vi "generate-uhd-class-lib.vi"() -> ()   [LabVIEW 2023]
panel:
  out "error out":errorcluster
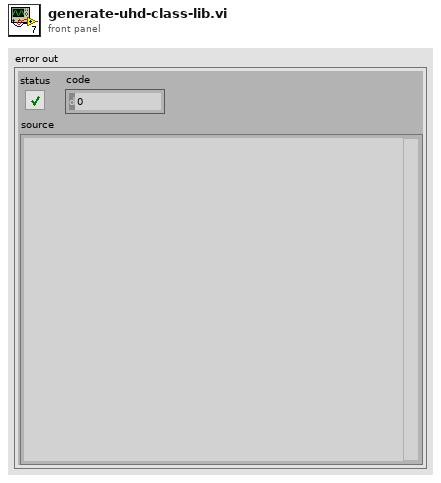
[diagram p1: front panel]
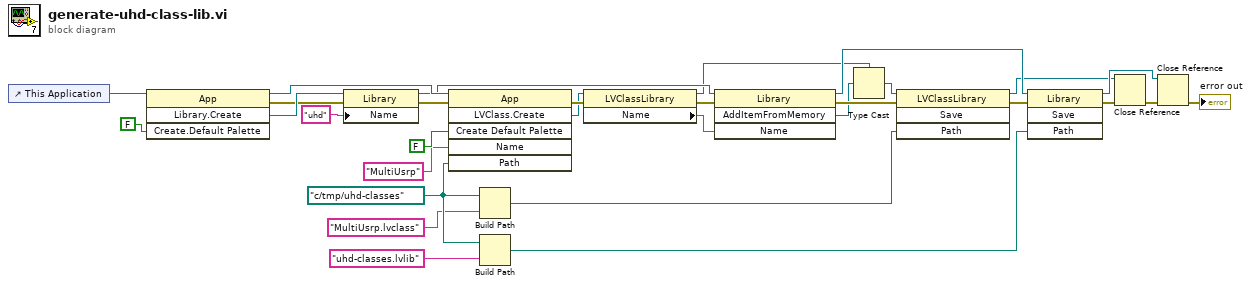
[diagram p0: block diagram]
diagram:
  w15 = path "c:/tmp/uhd-classes"
  n1 = control-ref of="This Application"() -> (w30:refnum<vi>)
  n2 = invoke class="App" method="Library.Create"(reference=w30, "Create.Default Palette"=FALSE ("Create:Default Palette")) -> (reference out=w28:refnum<vi>, error out=w21:errorcluster, "Create Library"=w23:refnum<vi>)  [unwired: 2 in, 1 out]
  n3 = property class="Library"(reference=w23, error in=w21, "Name"="uhd") -> (reference out=w13:refnum<vi>, error out=w20:errorcluster)
  n4 = invoke class="App" method="LVClass.Create"(reference=w28, error in=w20, "Create Default Palette"=FALSE ("Create:Default Palette"), "Name"="MultiUsrp", "Path"=w15) -> (error out=w11:errorcluster, "LVClass.Create"=w1:refnum<vi>)  [unwired: 1 in, 4 out]
  n5 = Build Path(base path=w15, name or relative path="MultiUsrp.lvclass" ("Name")) -> (appended path=w9:path)
  n6 = Build Path(base path=w15, name or relative path="uhd-classes.lvlib" ("Name")) -> (appended path=w16:path)
  n7 = property class="LVClassLibrary"(reference=w1, error in=w11) -> (reference out=w3:refnum<vi>, error out=w10:errorcluster, "Name"=w12:string)
  n8 = invoke class="Library" method="AddItemFromMemory"(reference=w13, error in=w10, "Name"=w12) -> (reference out=w6:refnum<vi>, error out=w8:errorcluster, "AddItemFromMemory"=w4:refnum<vi>)  [unwired: 1 in, 1 out]
  n9 = Type Cast(type=w3, x=w4) -> (*(type *) &x=w2:refnum<vi>)
  n10 = invoke class="LVClassLibrary" method="Save"(reference=w2, error in=w8, "Path"=w9) -> (reference out=w5:refnum<vi>, error out=w7:errorcluster)  [unwired: 1 in, 2 out]
  n11 = invoke class="Library" method="Save"(reference=w6, error in=w7, "Path"=w16) -> (reference out=w24:refnum<vi>, error out=w19:errorcluster)  [unwired: 1 in, 2 out]
  n12 = Close Reference(reference=w5, error in (no error)=w19) -> (error out=w18:errorcluster)
  n13 = Close Reference(reference=w24, error in (no error)=w18) -> (error out=→"error out":errorcluster)
